vi "RTS Parse Setup File.vi"(11 "Data":string) -> (1 "Save Path":path, 2 "Setup Info Station 8":string[][](array[string]), 3 "Station ID":string)   [LabVIEW 2020]
uses:
  Type Definitions/RTS TCP Commands.ctl
  <vilib>/Utility/error.llb/whitespace.ctl
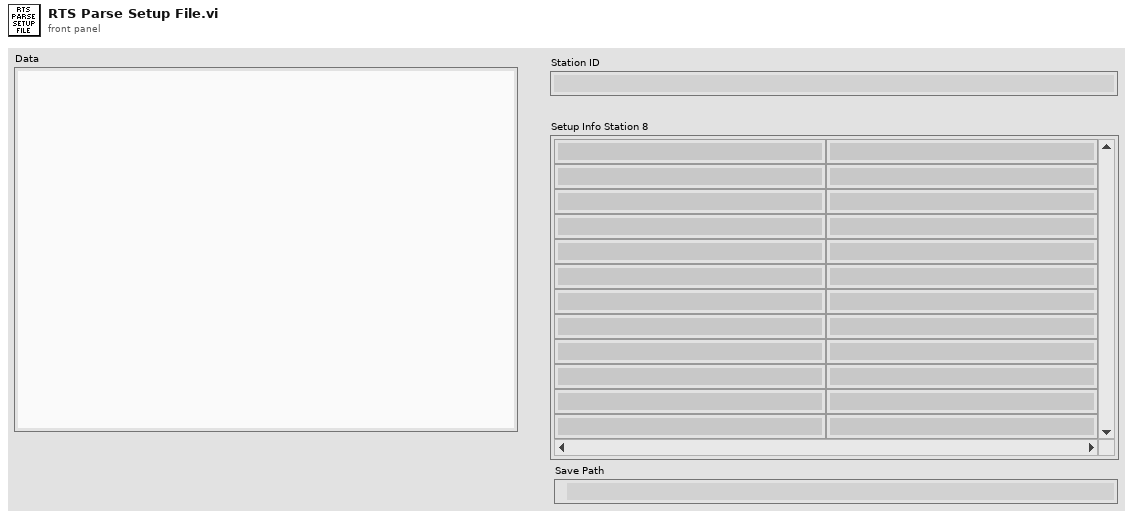
[diagram p1: front panel]
types:
  T1 = typedef "whitespace.ctl" = u16
  T2 = typedef "RTS TCP Commands.ctl" = string
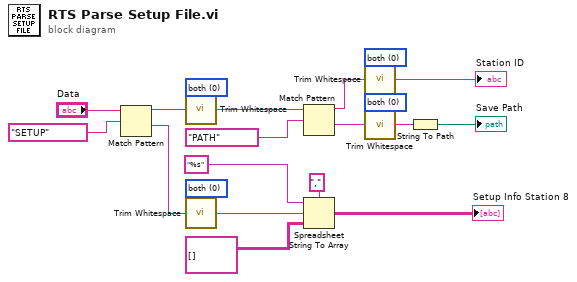
[diagram p0: block diagram]
diagram:
  w3 = T1 0 items=["both", "start of string", "end of string"] ("location (both)")
  w7 = T1 0 items=["both", "start of string", "end of string"] ("location (both)")
  w15 = T1 0 items=["both", "start of string", "end of string"] ("location (both)")
  w10 = T1 0 items=["both", "start of string", "end of string"] ("location (both)")
  n1 = Match Pattern(string="Data", regular expression=T2 "SETUP" ("TCP Commands")) -> (before substring=w12:string, after substring=w13:string)  [unwired: 1 in, 2 out]
  n2 = call <vilib>:"Trim Whitespace.vi"("string"=w12, "location (both)"=w15) -> ("trimmed string"=w8:string)
  n3 = call <vilib>:"Trim Whitespace.vi"("string"=w13, "location (both)"=w10) -> ("trimmed string"=w18:string)
  n4 = Match Pattern(string=w8, regular expression=T2 "PATH" ("TCP Commands")) -> (before substring=w6:string, after substring=w2:string)  [unwired: 1 in, 2 out]
  n5 = Spreadsheet String To Array(delimiter (Tab)=",", format string="%s", spreadsheet string=w18, array type (2D Dbl)=string[][] [] ("Setup Info Station 8")) -> (array=→"Setup Info Station 8":string[][])
  n6 = call <vilib>:"Trim Whitespace.vi"("string"=w6, "location (both)"=w7) -> ("trimmed string"=→"Station ID":string)
  n7 = call <vilib>:"Trim Whitespace.vi"("string"=w2, "location (both)"=w3) -> ("trimmed string"=w1:string)
  n8 = String To Path(string=w1) -> (path=→"Save Path":path)
